vi "Get Cal Manager.vi"(4 "현장리스트?":bool, 6 "인증교정자 참조":refnum<vi>, 8 "에러 입력(에러 없음)":errorcluster, 9 "기책사번":string, 10 "교정정보 in":T1, 11 "참조 번호 입력":T2) -> (0 "에러 출력":errorcluster, 2 "교정정보 out":T1, 3 "참조 번호 출력":T2)   [LabVIEW 2020]
uses:
  Controls/Clst_Cal Info Global.ctl
  <vilib>/addons/database/Connection.llb/Conn ObjectReference.ctl
  Controls/Cmd_Read Query.ctl
  Controls/Clst_Query Info.ctl
  Public/Polymorph/ini Ctrl_Str.vi
  <vilib>/addons/database/NI_Database_API.lvlib
panel:
  out "배열":string[](array[string])
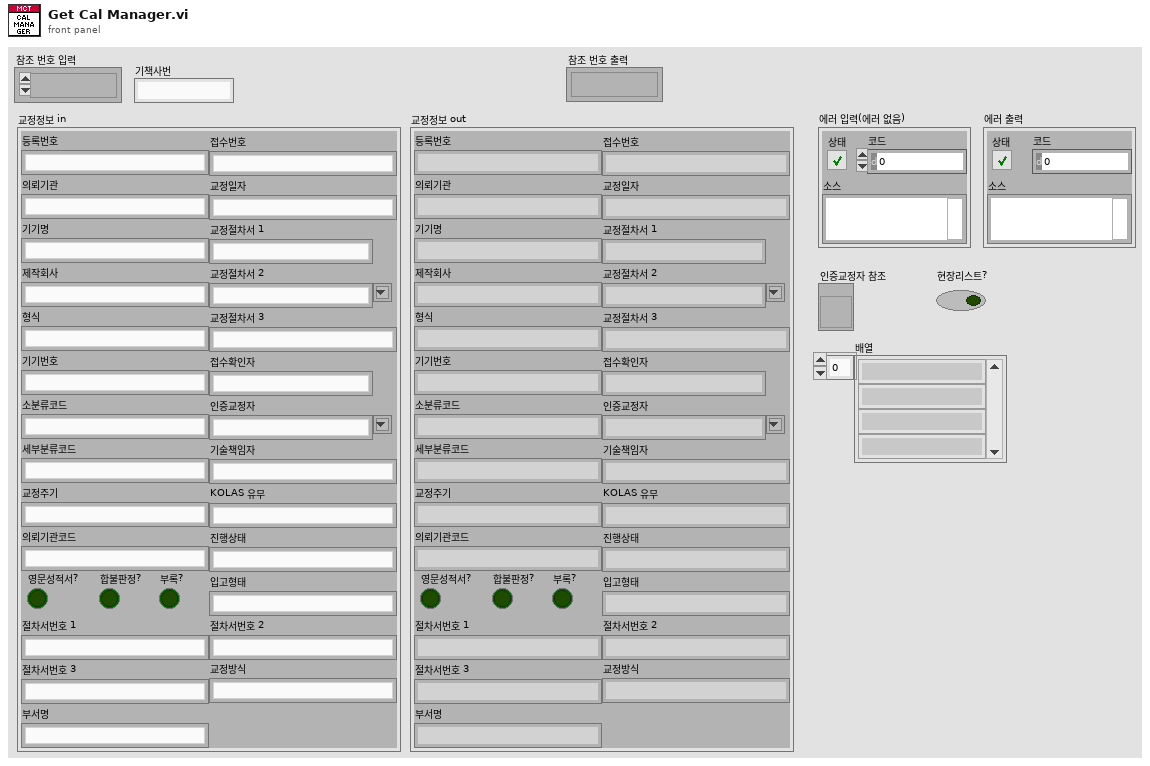
[diagram p1: front panel]
types:
  T1 = typedef "Clst_Cal Info Global.ctl" = cluster{"등록번호":string, "의뢰기관":string, "기기명":string, "제작회사":string, "형식":string, "기기번호":string, "소분류코드":string, "세부분류코드":string, "교정주기":string, "접수번호":string, "교정일자":string, "교정절차서 1":string, "교정절차서 2":string, "교정절차서 3":string, "접수확인자":string, "인증교정자":string, "기술책임자":string, "KOLAS 유무":string, "진행상태":string, "의뢰기관코드":string, "입고형태":string, "영문성적서?":bool, "합불판정?":bool, "부록?":bool, "절차서번호 1":string, "절차서번호 2":string, "절차서번호 3":string, "교정방식":string, "부서명":string}
  T2 = typedef "NI_Database_API.lvlib/Conn ObjectReference.ctl" = refnum<k1>
  T3 = typedef "Clst_Query Info.ctl" = cluster{"사번":string, "등록번호":string, "업체명":string, "세부분류코드":string, "형식":string, "기기번호":string, "FUNC":string, "FUNC_EXT":string, "옵션":string, "추가문자열":string, "일자":string, "배열 1":string[], "배열 2":string[], "항목명":string, "문자열":string, "이름":string}
  T4 = typedef "Cmd_Read Query.ctl" = enum16{"교정자 이름 얻기", "인증교정자 얻기", "기술책임자 얻기", "기책부책 얻기", "등록번호 얻기", "등록정보 얻기", "업체정보 얻기", "교정일자(CAMAS) 얻기", "교정일자(CALSTD) 얻기", "교정환경 얻기", "교정절차서 목록 얻기", "교정절차서명 얻기", "교정절차 목록얻기", "교정절차 얻기", "PROC 교정절차 얻기", "PROC SPEC 얻기", "교정절차(Func별) 얻기", "교정절차(Func_ext별) 얻기", "기관코드 얻기", "교정기능(세부분류) 얻기", "교정기능(모델) 얻기", "교정기능 목록 얻기", "교정기능 명칭 얻기", "교정기능 항목명칭 얻기", "DB (사용기준기) 얻기", "DB (기준기이름) 얻기", "DB (기준기이름목록) 얻기", "DB (기준기목록) 얻기", "DB (기준기값) 얻기", "DB (CMC) 얻기", "DB (FUNC) 얻기", "DB (CALNAME) 얻기", "DB (STDNAME) 얻기", "DB (SPEC) 얻기", "모델(항목전체) 얻기", "모델(최대범위) 얻기", "모델(최소범위) 얻기", "모델(최대최소) 얻기", "모델(범위조건) 얻기", "모델(등록요청) 얻기", "모델(형식별) 얻기", "모델(조건별) 얻기", "모델(모델검색) 얻기", "세부분류 목록 얻기", "기준기등록리스트 얻기", "STD Cal Date Check", "DB등록일자 얻기", "적용항목 얻기", "기타정보 얻기", "기준기요청 얻기", "서버버전 얻기"}
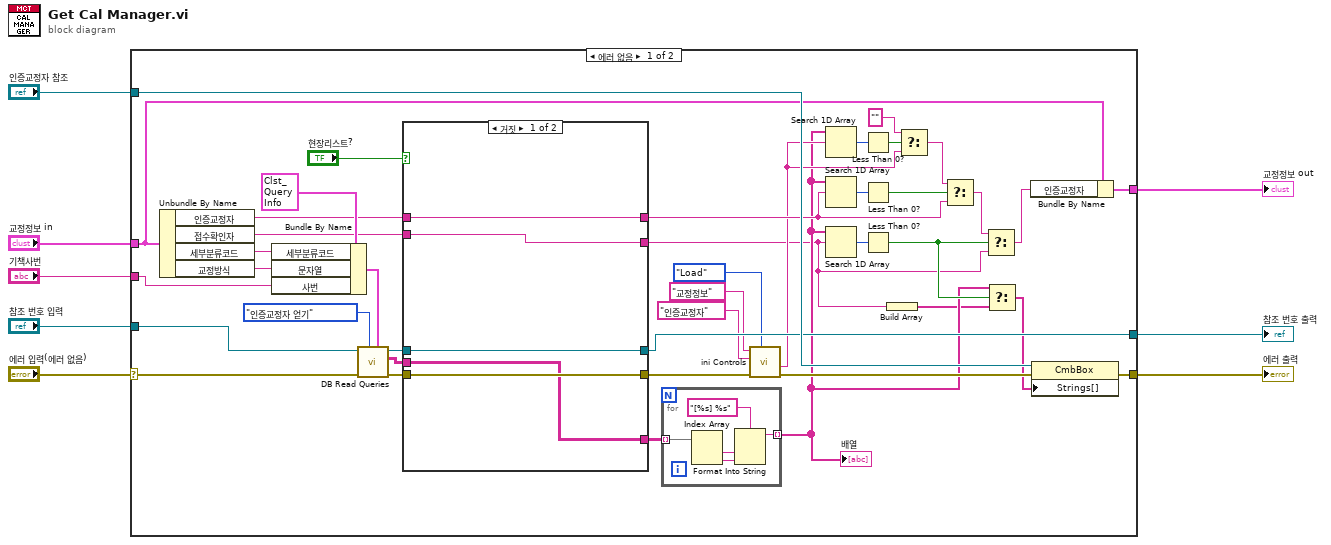
[diagram p0: block diagram]
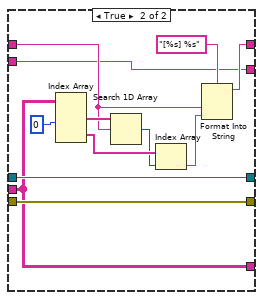
[diagram p2: hidden frame]
diagram:
  n1 = case shown="에러 없음" "에러 입력(에러 없음)" {
    selector: "에러 입력(에러 없음)" -> [w28 w74]
    tunnel: [w49 w74] -> w8
    tunnel: "인증교정자 참조" -> [w48 _]
    tunnel: "참조 번호 입력" -> [w45 w73]
    tunnel: [w44 w72] -> w5
    tunnel: "교정정보 in" -> [w43 w72]
    tunnel: [w37 w73] -> w3
    tunnel: "기책사번" -> [w10 _]
    frame No Error {
      n2 = Unbundle By Name(w43) -> ("인증교정자"=w33:string, "접수확인자"=w29:string, "세부분류코드"=w39:string, "교정방식"=w9:string)
      n3 = Bundle By Name(cluster=T3 {"사번"="", "등록번호"="", "업체명"="", "세부분류코드"="", "형식"="", "기기번호"="", "FUNC"="", "FUNC_EXT"="", "옵션"="", "추가문자열"="", "일자"="", "배열 1"=[], "배열 2"=[], "항목명"="", "문자열"="", "이름"=""} ("Query info"), "세부분류코드"=w39, "문자열"=w9, "사번"=w10) -> (w35:T3)
      n4 = call "DB Read Queries.vi"("Query info"=w35, "Query Command"=Cmd_Read_Query."인증교정자 얻기", "에러 입력(에러 없음)"=w28, "참조 번호 입력"=w45) -> ("에러 출력"=w36:errorcluster, "Data"=w31:string[][], "참조 번호 출력"=w38:T2)  [unwired: 3 in, 2 out]
      n5 = case shown="거짓" "현장리스트?" {
        tunnel: w38 -> [w52 w66]
        tunnel: [w52 w66] -> w37
        tunnel: w36 -> [w51 w65]
        tunnel: [w51 w65] -> w27
        tunnel: w33 -> [w54 w59]
        tunnel: [w54 w56] -> w32
        tunnel: w29 -> [w53 w55]
        tunnel: [w53 w55] -> w11
        tunnel: w31 -> [w50 w62]
        tunnel: [w50 w62] -> w30
        frame False {
        }
        frame True {
          n6 = Index Array(array=w62, index (col) #1=0 ("비활성화된 인덱스 (열)")) -> (element #1=w63:string[], element #2=w61:string[])  [unwired: 3 in]
          n7 = Search 1D Array(1D array=w63, element=w59) -> (index of element=w60:i32)  [unwired: 1 in]
          n8 = Index Array(array=w61, index=w60) -> (element=w58:string)
          n9 = Format Into String(format string="[%s] %s" ("포맷 문자열"), w59, w58) -> (resulting string=w56:string)  [unwired: 2 in, 1 out]
        }
      }
      n10 = for {
        tunnel: w30 -> [w70] mode=indexing
        tunnel: [w67] -> w13 mode=indexing
        n11 = Index Array(array=w70) -> (element #1=w69:string, element #2=w68:string)  [unwired: 2 in]
        n12 = Format Into String(format string="[%s] %s" ("포맷 문자열"), w69, w68) -> (resulting string=w67:string)  [unwired: 2 in, 1 out]
      }
      "배열" <- w13
      n13 = call-poly "ini Controls.vi"("Select"=enum16{"Save", "Load"}."Load", "에러 입력"=w27, "키"="인증교정자" ("key"), "섹션"="교정정보" ("section")) -> ("에러 출력"=w26:errorcluster, "값"=w18:string)  [unwired: 5 in, 1 out]
      n14 = Search 1D Array(1D array=w13, element=w18) -> (index of element=w22:i32)  [unwired: 1 in]
      n15 = Search 1D Array(1D array=w13, element=w32) -> (index of element=w40:i32)  [unwired: 1 in]
      n16 = Search 1D Array(1D array=w13, element=w11) -> (index of element=w42:i32)  [unwired: 1 in]
      n17 = Less Than 0?(x=w22) -> (x < 0?=w21:bool)
      n18 = Less Than 0?(x=w40) -> (x < 0?=w41:bool)
      n19 = Less Than 0?(x=w42) -> (x < 0?=w14:bool)
      n20 = Build Array(w11) -> (w12:string[])
      n21 = Select(t="", s=w21, f=w18) -> (s? t:f=w19:string)
      n22 = Select(t=w19, s=w41, f=w32) -> (s? t:f=w15:string)
      n23 = Select(t=w15, s=w14, f=w11) -> (s? t:f=w16:string)
      n24 = Select(t=w13, s=w14, f=w12) -> (s? t:f=w17:string[])
      n25 = Bundle By Name(cluster=w43, "인증교정자"=w16) -> (w44:T1)
      n26 = property class="CmbBox"(reference=w48, error in=w26, "Strings[]"=w17) -> (error out=w49:errorcluster)  [unwired: 1 out]
    }
    frame Error {
    }
  }
  "에러 출력" <- w8
  "참조 번호 출력" <- w3
  "교정정보 out" <- w5
